vi "Close.vi"(8 "error in":errorcluster) -> (0 "error out":errorcluster, 2 "result":bool)   [LabVIEW 2016]
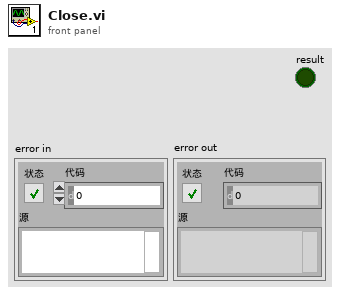
[diagram p1: front panel]
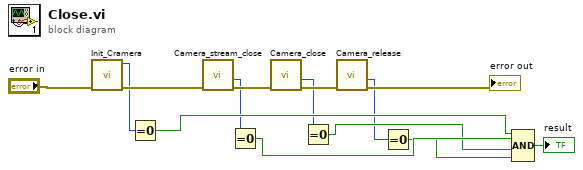
[diagram p0: block diagram]
diagram:
  n1 = call "Init_Cramera.vi"("error in"="error in") -> ("error out"=w10:errorcluster, "初始化返回值"=w1:i32)  [unwired: 9 in]
  n2 = Equal To 0?(x=w1) -> (x = 0?=w9:bool)
  n3 = call "Camera_stream_close.vi"("error in"=w10) -> ("error out"=w14:errorcluster, "关闭内部出图返回值"=w5:i32)  [unwired: 9 in]
  n4 = Equal To 0?(x=w5) -> (x = 0?=w8:bool)
  n5 = call "Camera_close.vi"("error in"=w14) -> ("error out"=w13:errorcluster, "关闭设备返回值"=w4:i32)  [unwired: 9 in]
  n6 = Equal To 0?(x=w4) -> (x = 0?=w7:bool)
  n7 = call "Camera_release.vi"("error in"=w13) -> ("error out"=→"error out":errorcluster, "释放资源返回值"=w3:i32)  [unwired: 9 in]
  n8 = Equal To 0?(x=w3) -> (x = 0?=w6:bool)
  n9 = Compound Arithmetic op=AND(w9, w8, w7, w6) -> (→"result":bool)
